vi "Replace Sweep Waveforms.vi"(10 "Channels New":T3 {"Table" format="%#_1f"; "Channel" min=1 max=128; "Start" format="%#_6p"; "End" format="%#_6p"}, 11 "Channels in":T3 {"Table" format="%#_1f"; "Channel" min=1 max=128; "Start" format="%#_6p"; "End" format="%#_6p"}) -> (3 "Channels out":T3 {"Table" format="%#_1f"; "Channel" min=1 max=128; "Start" format="%#_6p"; "End" format="%#_6p"})   [LabVIEW 2019, in "Instrument.Lockin.lvclass"]
uses:
  Instrument.Lockin.lvclass
  Instrument.DAQ/Typedefs/Sweep.Channel--Cluster--Array.ctl
  Instrument.DAQ/Typedefs/Sweep.Channel--Cluster.ctl
  Instrument.DAQ/Typedefs/Sweep.Pattern--Enum.ctl
  Instrument.DAQ/Instrument.DAQ.lvclass
panel:
  out "Array":T2(array[cluster])
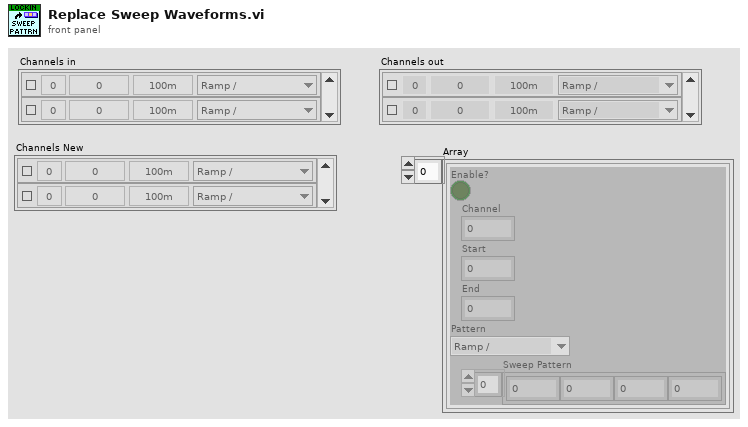
[diagram p1: front panel]
types:
  T1 = typedef "Instrument.DAQ.lvclass/Sweep.Pattern--Enum.ctl" = enum16{"Ramp /", "Ramp /\\", "Smooth Ramp _/", "Smooth Ramp _/\\_", "Table"}
  T2 = cluster{"Enable?":bool, "Channel":u16, "Start":dbl, "End":dbl, "Pattern":T1, "Sweep Pattern":dbl[]}[]
  T3 = typedef "Instrument.DAQ.lvclass/Sweep.Channel--Cluster--Array.ctl" = T4[]
  T4 = typedef "Instrument.DAQ.lvclass/Sweep.Channel--Cluster.ctl" = cluster{"Enable?":bool, "Channel":u16, "Start":dbl, "End":dbl, "Pattern":T1, "Table":dbl[]}
  T5 = cluster{"Enable?":bool, "Channel":u16, "Start":dbl, "End":dbl, "Pattern":T1, "Table":dbl[]}
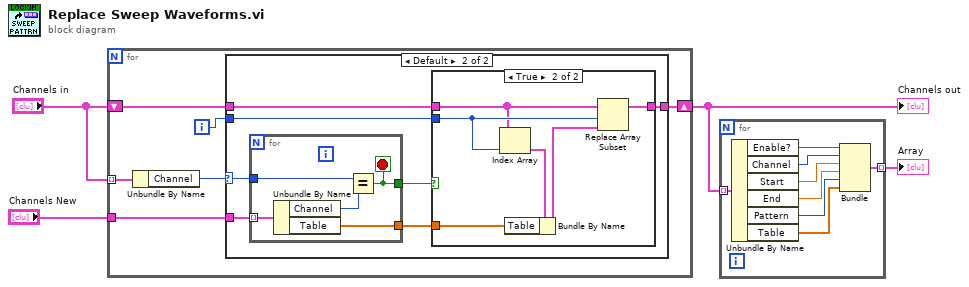
[diagram p0: block diagram]
diagram:
  n1 = for {
    tunnel: "Channels New" -> [w7]
    shift-right: [w10] -> w3
    shift-left: "Channels in" -> [w9]
    tunnel: "Channels in" -> [w8] mode=indexing
    i -> [w5]
    n2 = Unbundle By Name(w8) -> ("Channel"=w6:u16)
    n3 = case shown="Default" w6 {
      selector: w6 -> [_ w15]
      tunnel: [w11 w18] -> w10
      tunnel: w9 -> [w11 w17]
      tunnel: w7 -> [_ w14]
      tunnel: w5 -> [_ w13]
      frame 0 {
      }
      frame Default {
        n4 = for {
          tunnel: w15 -> [w21]
          tunnel: [w23] -> w16
          tunnel: w14 -> [w22] mode=indexing
          tunnel: [w19] -> w12
          stop <- w23 stop-if-true
          n5 = Unbundle By Name(w22) -> ("Channel"=w20:u16, "Table"=w19:dbl[])
          n6 = Equal?(x=w21, y=w20) -> (x = y?=w23:bool)
        }
        n7 = case shown="True" w16 {
          tunnel: w17 -> [w24 w25]
          tunnel: [w24 w30] -> w18
          tunnel: w13 -> [_ w29]
          tunnel: w12 -> [_ w27]
          frame False {
          }
          frame True {
            n8 = Index Array(array=w25, index=w29) -> (element=w28:T4)
            n9 = Bundle By Name(cluster=w28, "Table"=w27) -> (w26:T4)
            n10 = Replace Array Subset(array=w25, new element=w26, index=w29) -> (w30:T3)
          }
        }
      }
    }
  }
  "Channels out" <- w3
  n11 = for {
    tunnel: w3 -> [w38] mode=indexing
    tunnel: [w31] -> w2 mode=indexing
    n12 = Unbundle By Name(w38) -> ("Enable?"=w37:bool, "Channel"=w36:u16, "Start"=w35:dbl, "End"=w34:dbl, "Pattern"=w33:T1, "Table"=w32:dbl[])
    n13 = Bundle("Enable?"=w37, "Channel"=w36, "Start"=w35, "End"=w34, "Pattern"=w33, "Table"=w32) -> (w31:T5)  [unwired: 1 in]
  }
  "Array" <- w2
